vi "measure_slope.vi"(8 "temp":dbl=22.0, 9 "power peak":dbl, 10 "correction factor":dbl=1.0, 11 "XYGraph in":refnum<vi>) -> (1 "Numeric 3":dbl, 2 "Numeric 2":dbl, 3 "Numeric":dbl, 4 "Numeric 4":dbl)   [LabVIEW 2013]
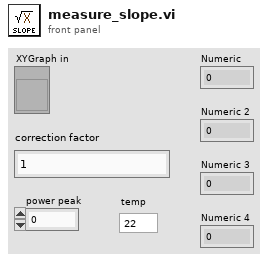
[diagram p1: front panel]
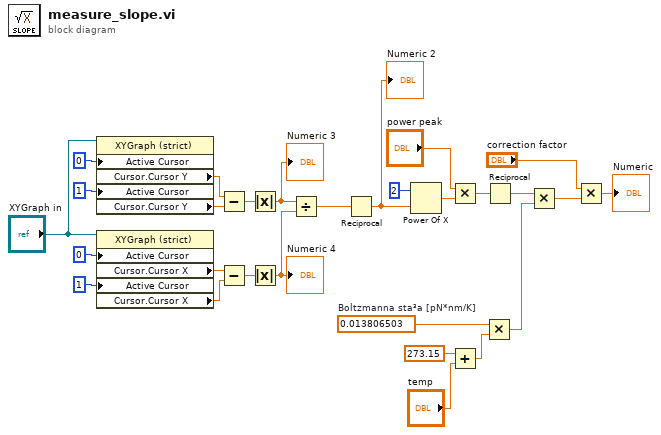
[diagram p0: block diagram]
diagram:
  w5 = 0.013806503  # Boltzmanna sta³a [pN*nm/K]
  n1 = property class="XYGraph (strict)"(reference="XYGraph in", "Active Cursor"=u32 0, "Active Cursor"=u32 1) -> ("Cursor.Cursor Y"=w17:dbl, "Cursor.Cursor Y"=w18:dbl)  [unwired: 1 in, 2 out]
  n2 = property class="XYGraph (strict)"(reference="XYGraph in", "Active Cursor"=u32 0, "Active Cursor"=u32 1) -> ("Cursor.Cursor X"=w14:dbl, "Cursor.Cursor X"=w15:dbl)  [unwired: 1 in, 2 out]
  n3 = Subtract(x=w17, y=w18) -> (x-y=w19:dbl)
  n4 = Subtract(x=w14, y=w15) -> (x-y=w16:dbl)
  n5 = Absolute Value(x=w19) -> (abs(x)=w8:dbl)
  "Numeric 3" <- w8
  n6 = Absolute Value(x=w16) -> (abs(x)=w6:dbl)
  "Numeric 4" <- w6
  n7 = Divide(x=w8, y=w6) -> (x/y=w7:dbl)
  n8 = Reciprocal(x=w7) -> (1/x=w9:dbl)
  "Numeric 2" <- w9
  n9 = Power Of X(1:w9, 2:2) -> (0:w20:dbl)
  n10 = Multiply(x="power peak", y=w20) -> (x*y=w24:dbl)
  n11 = Add(x=273.15 ("y"), y="temp") -> (x+y=w4:dbl)
  n12 = Multiply(x=w5, y=w4) -> (x*y=w2:dbl)
  n13 = Reciprocal(x=w24) -> (1/x=w22:dbl)
  n14 = Multiply(x=w22, y=w2) -> (x*y=w25:dbl)
  n15 = Multiply(x="correction factor", y=w25) -> (x*y=→"Numeric":dbl)
